vi "Write Actors Enqueuer.vi"(8 "error in (no error)":errorcluster, 10 "Actors Enqueuer":T1(c390), 11 "UIActorTop in":refnum<class "UIActorTop.lvclass">) -> (0 "error out":errorcluster, 3 "UIActorTop out":refnum<class "UIActorTop.lvclass">)   [LabVIEW 2021, in "AbstractActorTemplate.lvlib" / "UIActorTop.lvclass"]
uses:
  <userlib>/John_Lib/AbstractActorTemplate/AbstractActorTemplate/UIActorTop.lvclass
  <userlib>/John_Lib/AbstractActorTemplate/AbstractActorTemplate/UIActorTop.lvclass/UIActorTop.ctl
  <vilib>/ActorFramework/Message Enqueuer/Message Enqueuer.lvclass
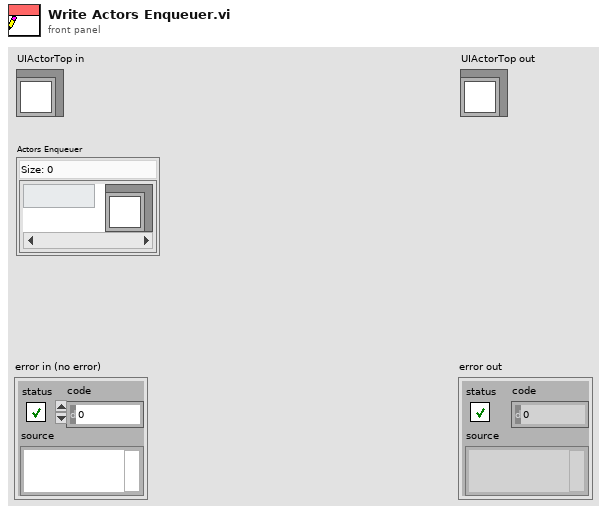
[diagram p1: front panel]
types:
  T1 = map{string, refnum<class "Message Enqueuer.lvclass">}
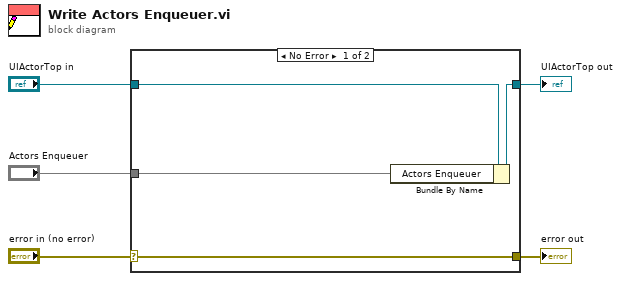
[diagram p0: block diagram]
diagram:
  n1 = case shown="No Error" "error in (no error)" {
    selector: "error in (no error)" -> [w9 w10]
    tunnel: [w9 w10] -> w4
    tunnel: [w7 w11] -> w2
    tunnel: "UIActorTop in" -> [w8 w11]
    tunnel: "Actors Enqueuer" -> [w6 _]
    frame No Error {
      n2 = Bundle By Name(cluster=w8, "Actors Enqueuer"=w6) -> (w7:refnum<class "UIActorTop.lvclass">)
    }
    frame Error {
    }
  }
  "error out" <- w4
  "UIActorTop out" <- w2
